vi "upg5_undersökstruktur.vi"() -> ()   [LabVIEW 2024]
panel:
  out "XY Graph":cluster{dbl[], "Mätvärden":dbl[]}(graph)
  in  "Mätvärden (m)":dbl[](array[numeric])
  out "radier (m)":dbl[](array[numeric])
  in  "A2 (m^2)":dbl
  out "dh/dt (m/s)":dbl[](array[numeric])
  in  "sampling frekvens: (Hz)":dbl=1.0 format="%0.2f"
  # "Kopiera in mätvärden"
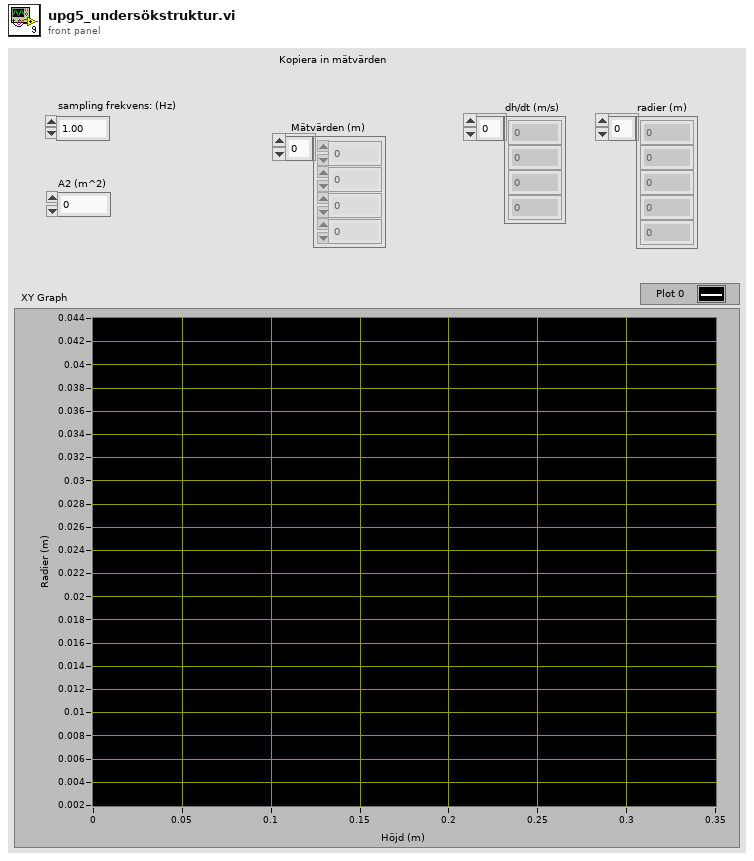
[diagram p1: front panel]
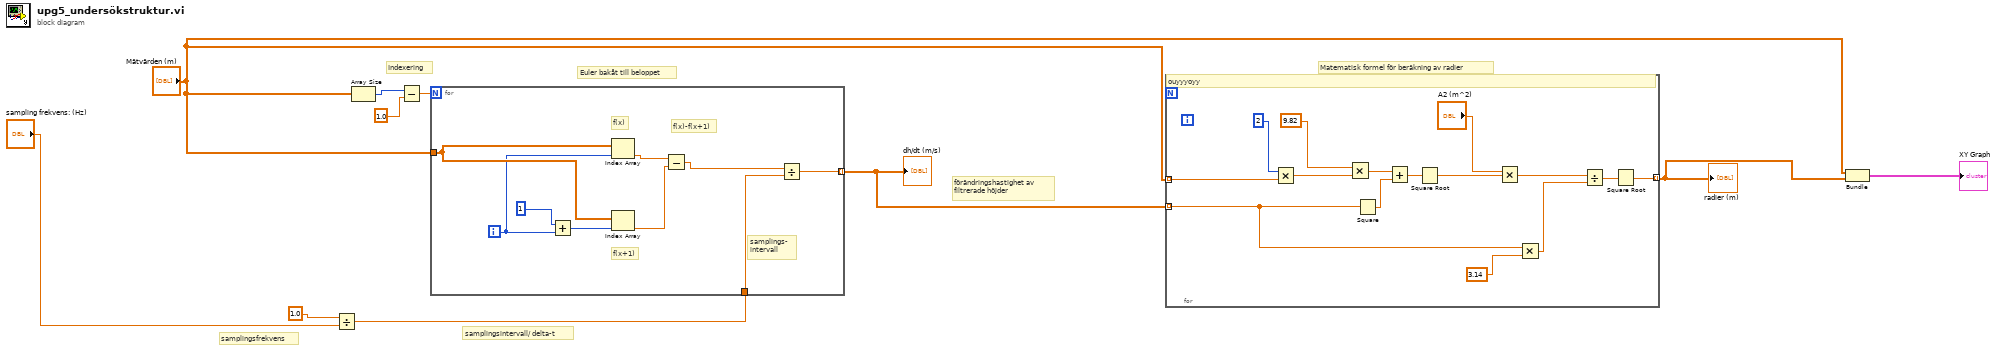
[diagram p0: block diagram]
diagram:
  # "Indexering"
  # "förändringshastighet av \nfiltrerade höjder"
  # "samplingsintervall/ delta-t"
  # "samplingsfrekvens"
  # "Matematisk formel för beräkning av radier"
  # "Euler bakåt till beloppet"
  n1 = Divide(x=1.0, y="sampling frekvens: (Hz)") -> (x/y=w7:dbl)
  n2 = Array Size(array="Mätvärden (m)") -> (size(s)=w4:i32)
  n3 = Subtract(x=w4, y=1.0) -> (x-y=w6:dbl)
  n4 = for {
    N: w6 -> [_]
    tunnel: "Mätvärden (m)" -> [w18]
    tunnel: [w16] -> w10 mode=indexing
    tunnel: w7 -> [w13]
    i -> [w14]
    # "samplings-\nintervall"
    # "f(x)-f(x+1)"
    # "f(x)"
    # "f(x+1)"
    n5 = Add(x=1, y=w14) -> (x+y=w19:i32)
    n6 = Index Array(array=w18, index=w14) -> (element=w12:dbl)
    n7 = Index Array(array=w18, index=w19) -> (element=w11:dbl)
    n8 = Subtract(x=w12, y=w11) -> (x-y=w17:dbl)
    n9 = Divide(x=w17, y=w13) -> (x/y=w16:dbl)
  }
  "dh/dt (m/s)" <- w10
  n10 = for {
    tunnel: w10 -> [w24] mode=indexing
    tunnel: "Mätvärden (m)" -> [w32] mode=indexing
    tunnel: [w26] -> w2 mode=indexing
    # "ouyyyoyy"
    n11 = Multiply(x=2, y=w32) -> (x*y=w33:dbl)
    n12 = Multiply(x=9.82, y=w33) -> (x*y=w30:dbl)
    n13 = Square(x=w24) -> (x^2=w31:dbl)
    n14 = Add(x=w30, y=w31) -> (x+y=w29:dbl)
    n15 = Square Root(x=w29) -> (sqrt(x)=w23:dbl)
    n16 = Multiply(x="A2 (m^2)", y=w23) -> (x*y=w21:dbl)
    n17 = Multiply(x=w24, y=3.14) -> (x*y=w28:dbl)
    n18 = Divide(x=w21, y=w28) -> (x/y=w27:dbl)
    n19 = Square Root(x=w27) -> (sqrt(x)=w26:dbl)
  }
  "radier (m)" <- w2
  n20 = Bundle("Mätvärden (m)"="Mätvärden (m)", w2) -> (→"XY Graph":cluster{"Mätvärden (m)":dbl[], dbl[]})  [unwired: 1 in]
